vi "Untitled 5.vi"() -> ()   [LabVIEW 2016]
panel:
  out "before substring":string
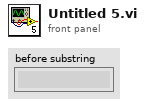
[diagram p1: front panel]
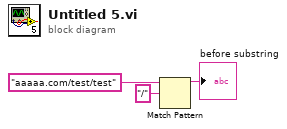
[diagram p0: block diagram]
diagram:
  n1 = Match Pattern(string="aaaaa.com/test/test", regular expression="/") -> (before substring=→"before substring":string)  [unwired: 1 in, 3 out]
